vi "Data Access.vi"(8 "error in (no error)":errorcluster, 10 "Data Access Handler":refnum<class "Data Access Handler.lvclass">, 11 "DMM Config Trigger Msg in":refnum<class "DMM Config Trigger Msg.lvclass">) -> (0 "error out":errorcluster, 3 "DMM Config Trigger Msg out":refnum<class "DMM Config Trigger Msg.lvclass">)   [LabVIEW 2020, in "DMM Msg.lvlib" / "DMM Config Trigger Msg.lvclass"]
doc: "Expose class private data to the front panel while letting the Data Access Handler class act on the data."
uses:
  DMM Config Trigger Msg.lvclass
  C:/Current projects/WS/PPL/HDH.Actor Framework.Core.Msg.lvlibp/Flex Msg/Flex Msg.lvclass
  PPL/HDH.Actor Framework.Core.Msg.lvlibp/Flex Msg/Data Access Handlers/Data Access Handler/Data Access Handler.lvclass
  PPL/HDH.Actor Framework.Core.Publisher.lvlibp/Messages/Response Msg/Response Core/Controls/Ctl_SendFunction.ctl
  DMM Config Trigger Msg.lvclass/DMM Config Trigger Msg.ctl
  PPL/HDH.Actor Framework.Core.Instrument Handler.lvlibp/Messages/Instrument Msg/Instrument Msg.lvclass
  C:/Current projects/WS/PPL/HDH.Actor Framework.Core.Instrument Handler.lvlibp/Messages/Instrument Msg/Instrument Msg.lvclass
  PPL/HDH.Actor Framework.Core.Publisher.lvlibp
panel:
  in  "Sample Interval(s)":dbl=-1.0 caption="Sample Interval (-1s)" format="%.2f"
  in  "Trigger Type Index":u16 caption="Trigger Type Index(0)"
  in  "Samples per Trigger":i32=1 caption="Samples per Trigger(1)"
  in  "Triggers to measure":i32=1 caption="Triggers to measure(1)"
  in  "Message Priority":enum16{"Low", "Normal", "High"}(ring)=enum."Normal"
  in  "Timeout if Waiting":i32=-1
  in  "Send Function":T1=enum."Await Reply"
  in  "Cancel":bool
  in  "OK":bool
  # "Send details"
  # "Configuration details"
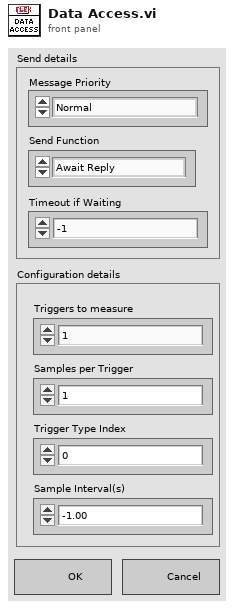
[diagram p1: front panel]
types:
  T1 = typedef "HDH.Actor Framework.Core.Publisher.lvlibp/Ctl_SendFunction.ctl" = enum16{"Send and Forget", "Request Reply", "Await Reply"}
  T2 = typedef "HDH.Actor Framework.Core.Actor.lvlibp/Message Enqueuer.lvclass/Message Priority.ctl" = enum16{"Low", "Normal", "High"}
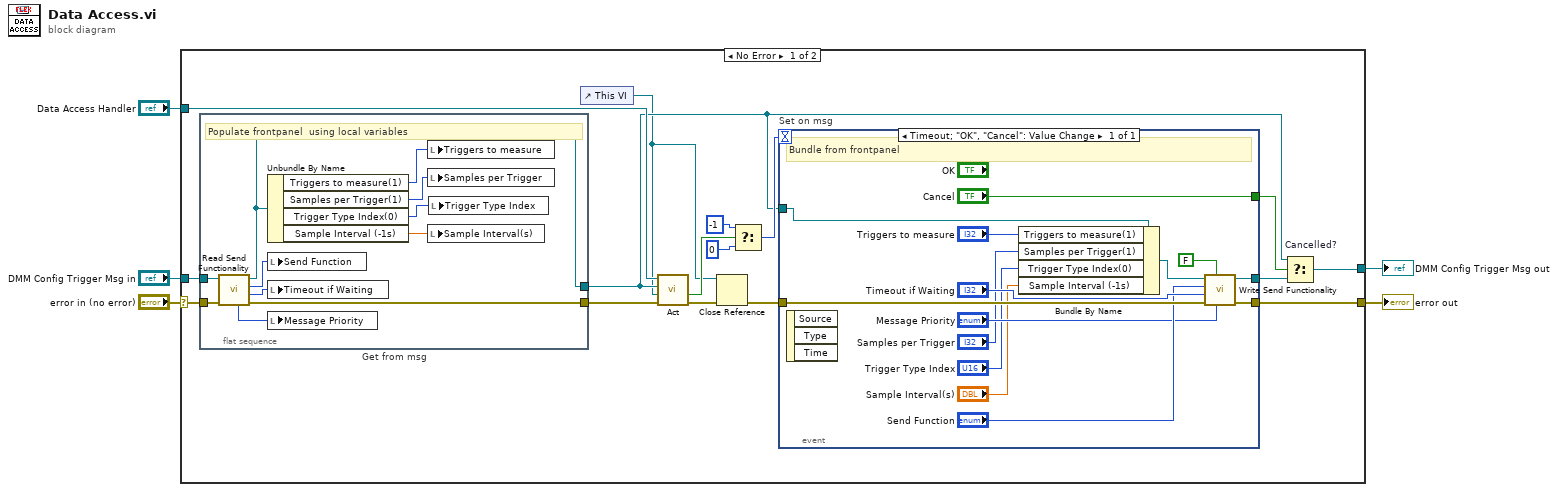
[diagram p0: block diagram]
diagram:
  n1 = case shown="No Error" "error in (no error)" {
    selector: "error in (no error)" -> [w21 w48]
    tunnel: [w14 w48] -> w4
    tunnel: [w9 w47] -> w2
    tunnel: "DMM Config Trigger Msg in" -> [w12 w47]
    tunnel: "Data Access Handler" -> [w20 _]
    frame No Error {
      n2 = flat-sequence "Get from msg" {
        tunnel: w21 -> [w45]
        tunnel: [w43] -> w7
        tunnel: w12 -> [w46]
        tunnel: [w44] -> w19
        frame #0 {
          # "Populate frontpanel  using local variables"
          n3 = call "Read Send Functionality.vi"("error in (no error)"=w45, "Instrument Msg in"=w46) -> ("error out"=w44:errorcluster, "Timeout if Waiting"=w41:i32, "Send Function"=w42:T1, "Instrument Msg out"=w43:refnum<class "DMM Config Trigger Msg.lvclass">, "Message Priority"=w40:T2)  [unwired: 4 in, 1 out]
          n4 = Unbundle By Name(w43) -> ("Triggers to measure(1)"=w39:i32, "Samples per Trigger(1)"=w38:i32, "Trigger Type Index(0)"=w37:u16, "Sample Interval (-1s)"=w36:dbl)
          n5 = local write "Send Function"(w42) -> ()
          n6 = local write "Timeout if Waiting"(w41) -> ()
          n7 = local write "Message Priority"(w40) -> ()
          n8 = local write "Triggers to measure"(w39) -> ()
          n9 = local write "Samples per Trigger"(w38) -> ()
          n10 = local write "Sample Interval(s)"(w36) -> ()
          n11 = local write "Trigger Type Index"(w37) -> ()
        }
      }
      n12 = control-ref of="This VI"() -> (w6:refnum<vi>)
      n13 = call-dynamic "Act.vi"("error in (no error)"=w19, "VI Refnum in"=w6, "Flex Msg type"=w7, "Data Access Handler in"=w20) -> ("error out"=w11:errorcluster, "Await user action?"=w18:bool)  [unwired: 5 in, 1 out]
      n14 = Close Reference(reference=w6, error in (no error)=w11) -> (error out=w13:errorcluster)
      n15 = Select(t=-1, s=w18, f=0 ("t")) -> (s? t:f=w15:i32)
      n16 = event "Set on msg" shown="[0] Timeout;  \"OK\", \"Cancel\": Value Change" {
        selector: _ -> [_]
        dyn-events: _ -> [_]
        timeout: w15 -> [_]
        tunnel: [w30] -> w14
        tunnel: w13 -> [w31]
        tunnel: ["Cancel"] -> w10
        tunnel: [w33] -> w8
        tunnel: w7 -> [w34]
        event Timeout; "OK", "Cancel": Value Change {
          # "Bundle from frontpanel"
          n17 = event-data() -> ()  [unwired: 1 in, 3 out]
          n18 = Bundle By Name(cluster=w34, "Triggers to measure(1)"="Triggers to measure", "Samples per Trigger(1)"="Samples per Trigger", "Trigger Type Index(0)"="Trigger Type Index", "Sample Interval (-1s)"="Sample Interval(s)") -> (w32:refnum<class "DMM Config Trigger Msg.lvclass">)
          n19 = call "Write Send Functionality.vi"("Message Priority(Normal)"="Message Priority", "Publish Data?(T)"=FALSE, "error in (no error)"=w31, "Timeout if Waiting(-1ms)"="Timeout if Waiting", "Send Function(Await Reply)"="Send Function", "Instrument Msg in"=w32) -> ("error out"=w30:errorcluster, "Instrument Msg out"=w33:refnum<class "DMM Config Trigger Msg.lvclass">)  [unwired: 4 in]
        }
      }
      n20 = Select "Cancelled?"(t=w7, s=w10, f=w8) -> (s? t:f=w9:refnum<class "DMM Config Trigger Msg.lvclass">)
    }
    frame Error {
    }
  }
  "error out" <- w4
  "DMM Config Trigger Msg out" <- w2
